vi "PROIECT3.vi"() -> ()   [LabVIEW 2021]
panel:
  out "COLD":bool
  out "MEDIUM":bool
  out "HOT":bool
  out "Thermometer":dbl(slide) scale=0.0..100.0
  out "u,y,r":cluster{"y":dbl, "u":dbl, "r-Set point":dbl}(graph)={"y"=4.981818181818582, "u"=4.98181818182085, "r-Set point"=4.9818181818181815}
  out "Comanda":dbl(slide)=4.981818181818582 scale=10.0..60.0
  in  "Referinta":dbl(slide)=50.10909090909091 scale=10.0..60.0
  in  "Kd":dbl(slide)=0.10101010101010102 scale=0.0..0.5
  in  "Ki":dbl(slide)=0.9090909090909092 scale=0.0..2.0
  in  "Kp":dbl(slide)=0.4292929292929293 scale=0.0..2.5
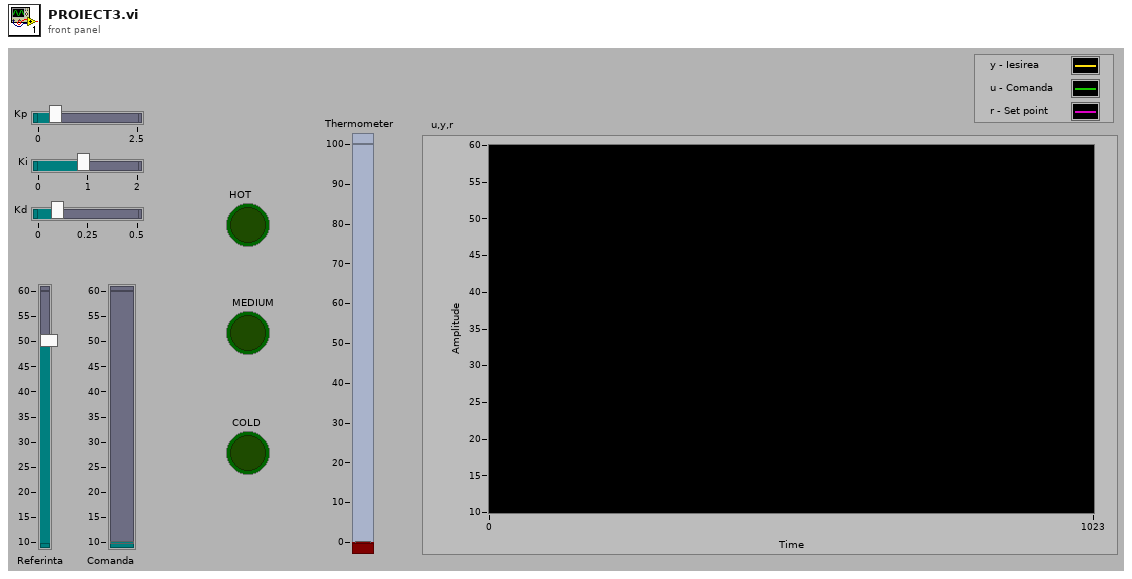
[diagram p1: front panel]
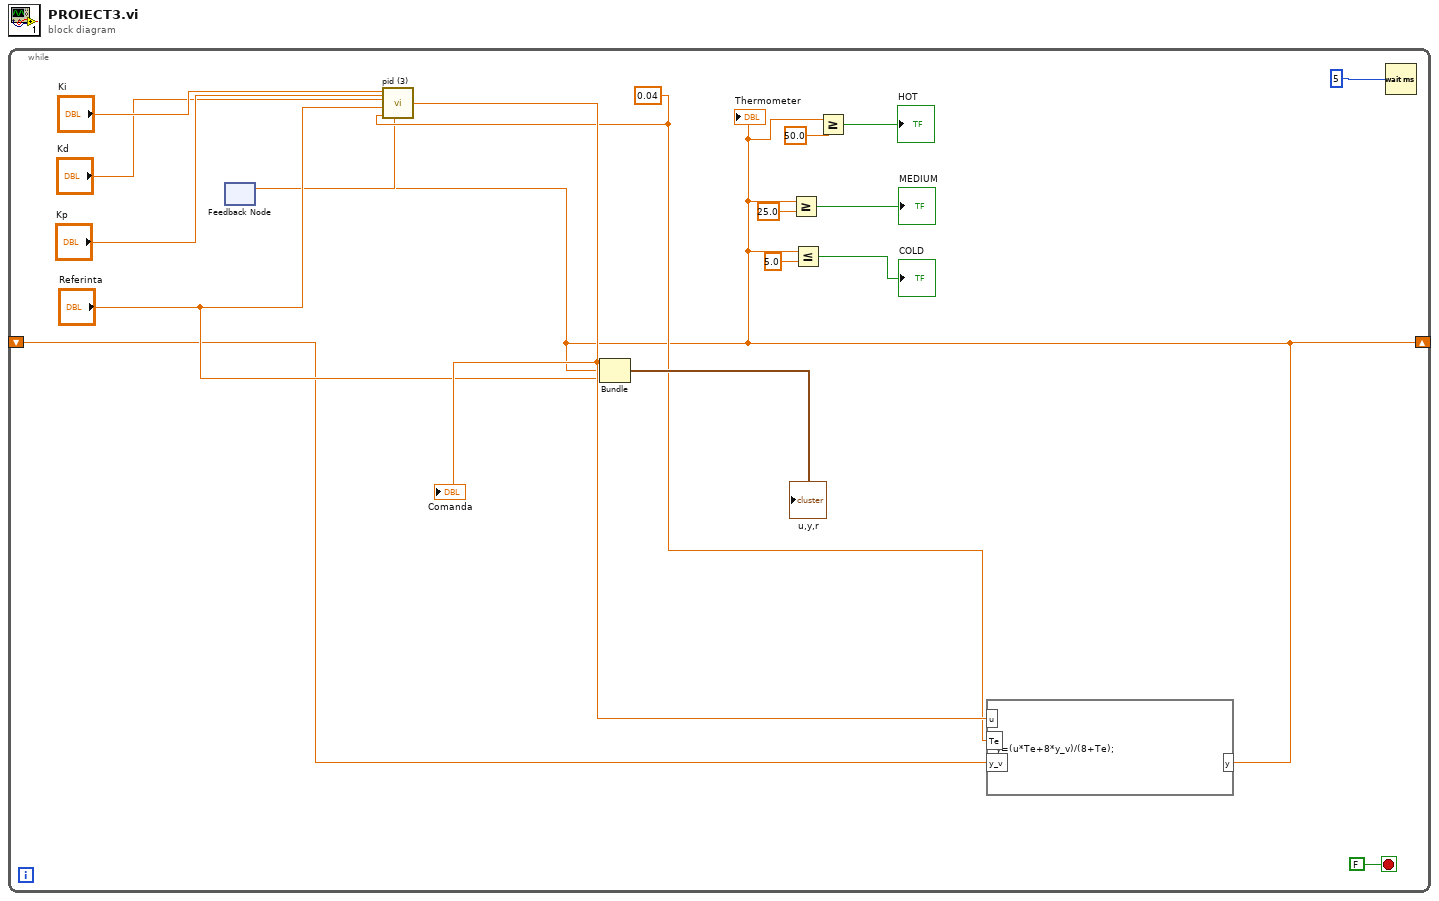
[diagram p0: block diagram]
diagram:
  n1 = while {
    shift-right: [w5] -> _
    shift-left: _ -> [w9]
    stop <- FALSE stop-if-true
    w11 = 0.04 ("Te")
    n2 = feedback #1() -> (w8:dbl)  [unwired: 1 in]
    n3 = call "pid (3).vi"("y"=w8, "Kp"="Kp", "Te"=w11, "r-Set point"="Referinta", "Kd"="Kd", "Ki"="Ki") -> ("u"=w14:dbl)
    "Comanda" <- w14
    n4 = formula code="y=(u*Te+8*y_v)/(8+Te);"("u"=w14, "Te"=w11, "y_v"=w9) -> ("y"=w5:dbl)
    "Thermometer" <- w5
    n5 = feedback-in #1(w5) -> ()
    n6 = Bundle("u"=w14, "y"=w5, "Referinta"="Referinta") -> (→"u,y,r":cluster{"u":dbl, "y":dbl, "Referinta":dbl})  [unwired: 1 in]
    n7 = Greater Or Equal?(x=w5, y=25.0) -> (x >= y?=→"MEDIUM":bool)
    n8 = Less Or Equal?(x=w5, y=5.0) -> (x <= y?=→"COLD":bool)
    n9 = Greater Or Equal?(x=w5, y=50.0) -> (x >= y?=→"HOT":bool)
    n10 = Wait (ms)(milliseconds to wait=u32 5) -> ()  [unwired: 1 out]
  }
